vi "XLP80_Action_InitWriteB.vi"(8 "err in":errorcluster) -> (0 "err out":errorcluster)   [LabVIEW 2021]
uses:
  XLP80_State_V001.llb/XLP80_State_TDefEnumGlobalState.ctl
  XLP80_Globals/Globals_Settings_XLP80.vi
  XLP80_Globals/XLP80_Globals_Referenzen.vi
  XLP80_Globals/XLP80_CAN_Globals.vi
panel:
  out "Index HV&Software":i32[](array[numeric])
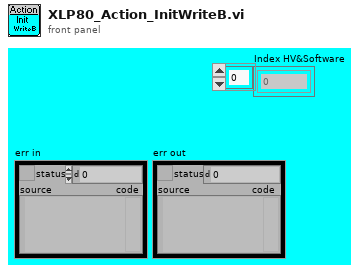
[diagram p1: front panel]
types:
  T1 = typedef "XLP80_State_TDefEnumGlobalState.ctl" = enum16{"HV & Software", "Basis Funktion", "Power Management", "Operational Mode", "Shutdown", "Alarm"}
  T2 = cluster{"Signal Name":string[], "Description":string[], "Unit":string[], "Default":dbl[], "Min":dbl[], "Max":dbl[], "Preconditions":bool[], "HV & Software":bool[], "Basis Funktion":bool[], "Power Management":bool[], "OperationMode":bool[], "Shutdown":bool[], "Alarm":bool[], "LogEnable":bool[]}
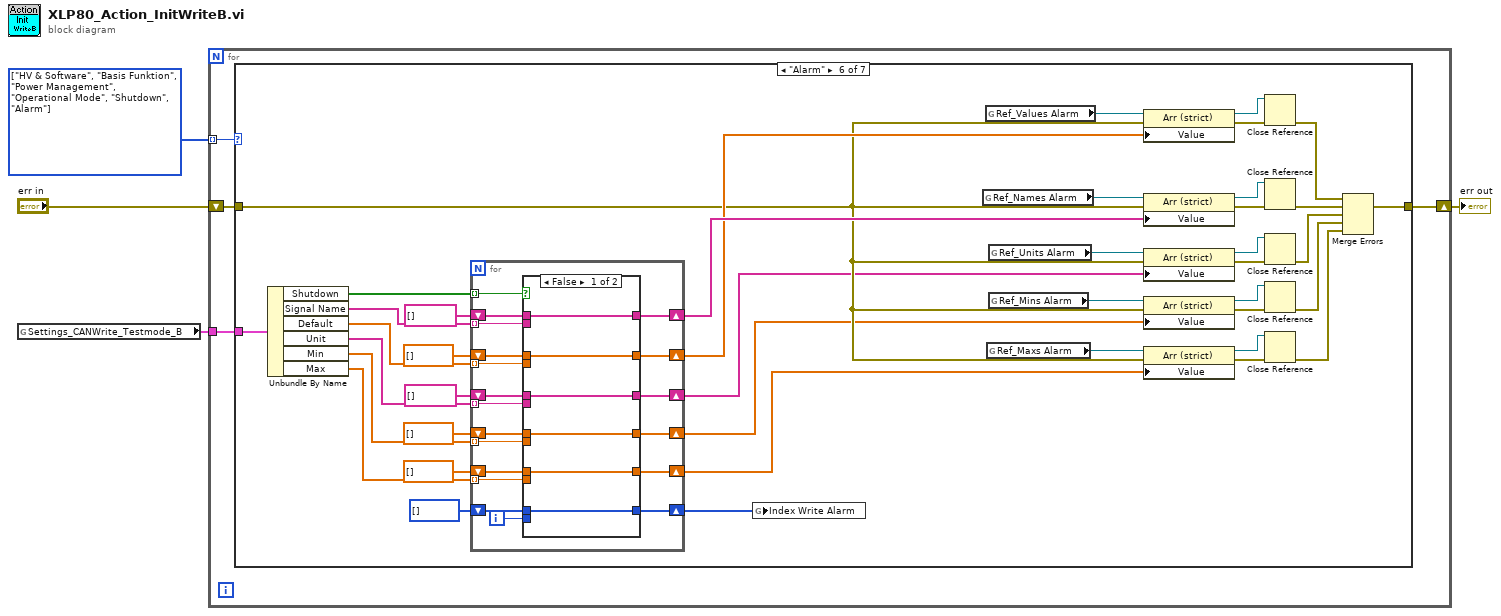
[diagram p0: block diagram]
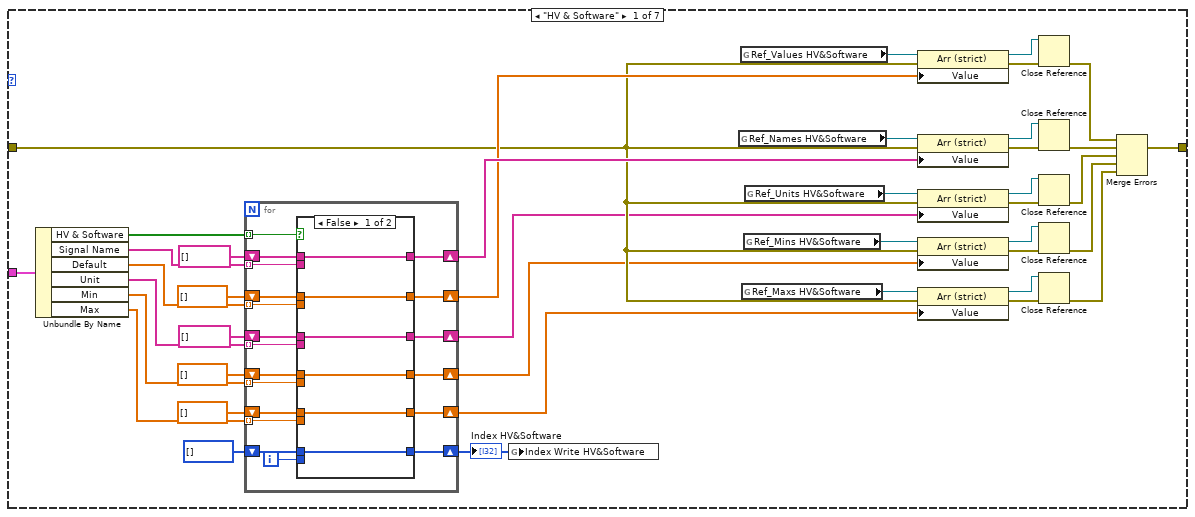
[diagram p2: hidden frame]
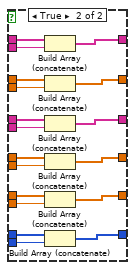
[diagram p3: hidden frame]
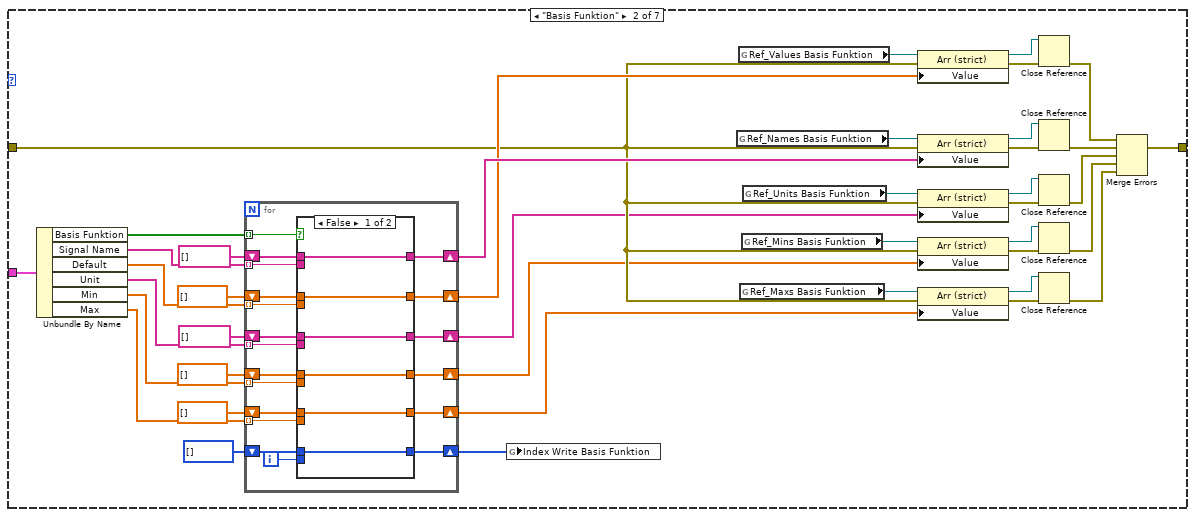
[diagram p4: hidden frame]
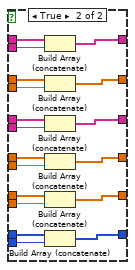
[diagram p5: hidden frame]
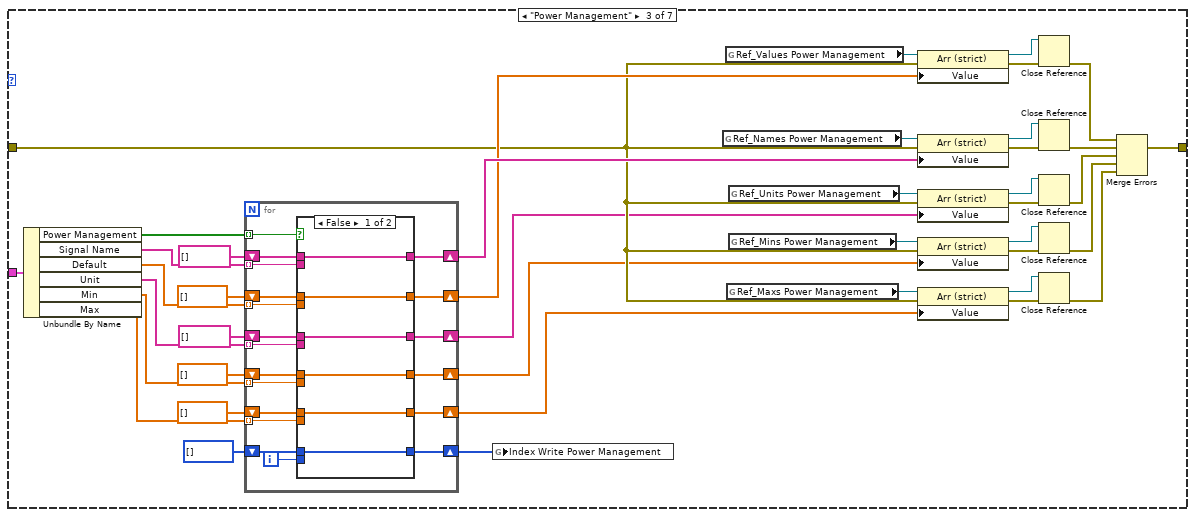
[diagram p6: hidden frame]
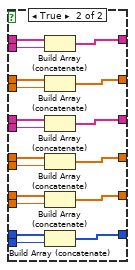
[diagram p7: hidden frame]
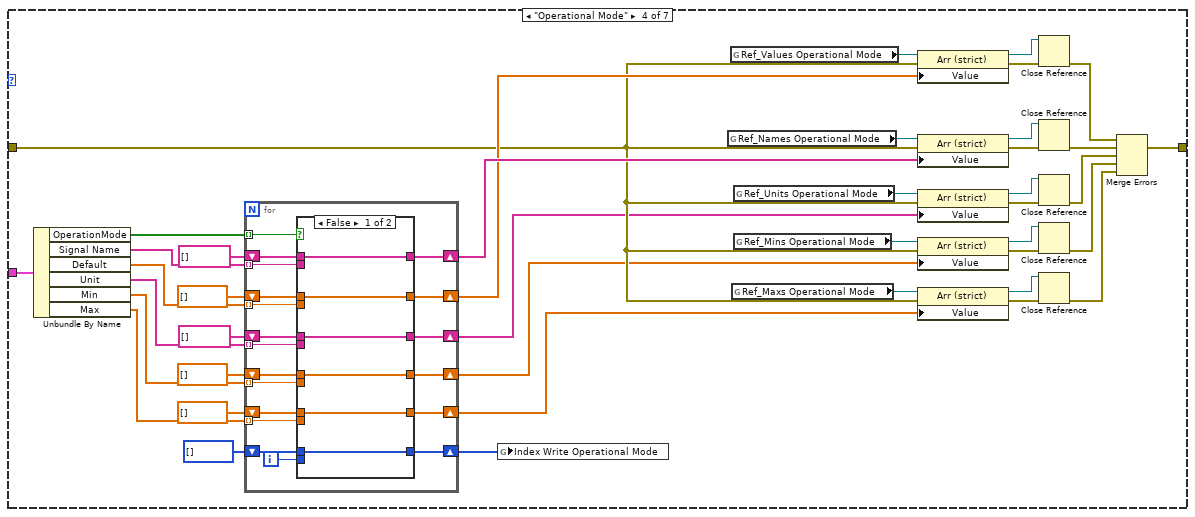
[diagram p8: hidden frame]
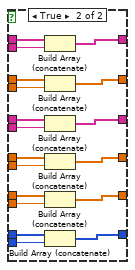
[diagram p9: hidden frame]
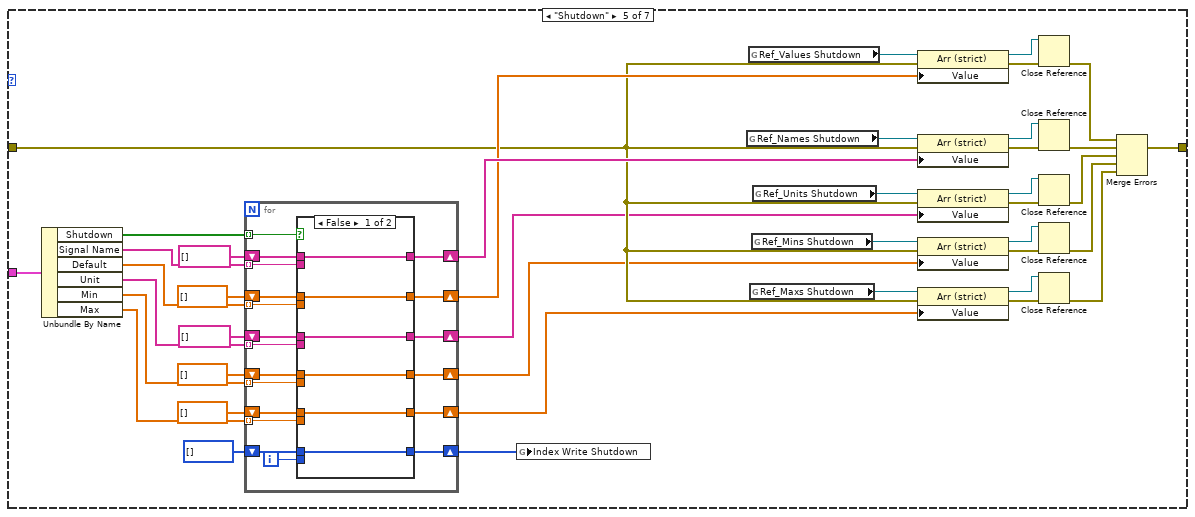
[diagram p10: hidden frame]
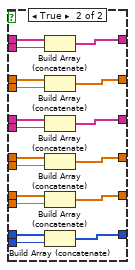
[diagram p11: hidden frame]
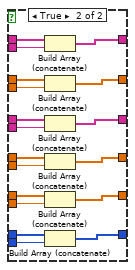
[diagram p12: hidden frame]
diagram:
  w1 = T1[] [enum."HV & Software", enum."Basis Funktion", enum."Power Management", enum."Operational Mode", enum."Shutdown", enum."Alarm"] items=["HV & Software", "Basis Funktion", "Power Management", "Operational Mode", "Shutdown", "Alarm"]
  n1 = global read "Globals_Settings_XLP80.vi" "Settings_CANWrite_Testmode_B"() -> (w4:T2)
  n2 = for {
    tunnel: w4 -> [w8]
    shift-right: [w6] -> w2
    shift-left: "err in" -> [w7]
    tunnel: w1 -> [w5] mode=indexing
    n3 = case shown="\"Alarm\"" w5 {
      tunnel: w8 -> [w49 w133 w217 w301 w385 w469 _]
      tunnel: w7 -> [w15 w99 w183 w267 w351 w435 w513]
      tunnel: [w35 w119 w203 w287 w371 w455 w513] -> w6
      frame "HV & Software" {
        n4 = Unbundle By Name(w49) -> ("HV & Software"=w40:bool[], "Signal Name"=w43:string[], "Default"=w32:dbl[], "Unit"=w27:string[], "Min"=w26:dbl[], "Max"=w25:dbl[])
        n5 = for {
          tunnel: w40 -> [w68] mode=indexing
          shift-right: [w65] -> w39
          shift-left: string[] [] ("Signal Name") -> [w67]
          shift-right: [w62] -> w41
          shift-left: i32[] [] -> [w64]
          tunnel: w43 -> [w66] mode=indexing
          shift-right: [w59] -> w31
          shift-left: dbl[] [] ("Default") -> [w61]
          tunnel: w32 -> [w60] mode=indexing
          shift-right: [w58] -> w10
          shift-left: dbl[] [] ("Default") -> [w56]
          tunnel: w26 -> [w57] mode=indexing
          shift-right: [w53] -> w9
          shift-left: dbl[] [] ("Default") -> [w55]
          tunnel: w25 -> [w54] mode=indexing
          shift-right: [w52] -> w11
          shift-left: string[] [] ("Signal Name") -> [w50]
          tunnel: w27 -> [w51] mode=indexing
          i -> [w63]
          n6 = case shown="False" w68 {
            tunnel: w67 -> [w74 w92]
            tunnel: w66 -> [_ w91]
            tunnel: [w74 w90] -> w65
            tunnel: w64 -> [w73 w89]
            tunnel: w63 -> [_ w88]
            tunnel: [w73 w87] -> w62
            tunnel: w61 -> [w72 w86]
            tunnel: w60 -> [_ w85]
            tunnel: [w72 w84] -> w59
            tunnel: w56 -> [w70 w81]
            tunnel: w57 -> [_ w82]
            tunnel: [w70 w83] -> w58
            tunnel: w55 -> [w69 w80]
            tunnel: w54 -> [_ w79]
            tunnel: [w69 w78] -> w53
            tunnel: w50 -> [w71 w75]
            tunnel: w51 -> [_ w76]
            tunnel: [w71 w77] -> w52
            frame False {
            }
            frame True {
              n7 = Build Array (concatenate)(w92, w91) -> (w90:string[])
              n8 = Build Array (concatenate)(w86, w85) -> (w84:dbl[])
              n9 = Build Array (concatenate)(w75, w76) -> (w77:string[])
              n10 = Build Array (concatenate)(w81, w82) -> (w83:dbl[])
              n11 = Build Array (concatenate)(w80, w79) -> (w78:dbl[])
              n12 = Build Array (concatenate)(w89, w88) -> (w87:i32[])
            }
          }
        }
        "Index HV&Software" <- w41
        n13 = global write "XLP80_CAN_Globals.vi" "Index Write HV&Software"(w41) -> ()
        n14 = global read "XLP80_Globals_Referenzen.vi" "Ref_Names HV&Software"() -> (w46:refnum<vi>)
        n15 = global read "XLP80_Globals_Referenzen.vi" "Ref_Values HV&Software"() -> (w36:refnum<vi>)
        n16 = global read "XLP80_Globals_Referenzen.vi" "Ref_Maxs HV&Software"() -> (w16:refnum<vi>)
        n17 = global read "XLP80_Globals_Referenzen.vi" "Ref_Mins HV&Software"() -> (w21:refnum<vi>)
        n18 = global read "XLP80_Globals_Referenzen.vi" "Ref_Units HV&Software"() -> (w24:refnum<vi>)
        n19 = property class="Arr (strict)"(reference=w36, error in=w15, "Value"=w31) -> (reference out=w38:refnum<vi>, error out=w37:errorcluster)
        n20 = property class="Arr (strict)"(reference=w46, error in=w15, "Value"=w39) -> (reference out=w47:refnum<vi>, error out=w48:errorcluster)
        n21 = property class="Arr (strict)"(reference=w24, error in=w15, "Value"=w11) -> (reference out=w22:refnum<vi>, error out=w23:errorcluster)
        n22 = property class="Arr (strict)"(reference=w21, error in=w15, "Value"=w10) -> (reference out=w20:refnum<vi>, error out=w19:errorcluster)
        n23 = property class="Arr (strict)"(reference=w16, error in=w15, "Value"=w9) -> (reference out=w17:refnum<vi>, error out=w18:errorcluster)
        n24 = Close Reference(reference=w38, error in (no error)=w37) -> (error out=w34:errorcluster)
        n25 = Close Reference(reference=w47, error in (no error)=w48) -> (error out=w45:errorcluster)
        n26 = Close Reference(reference=w22, error in (no error)=w23) -> (error out=w14:errorcluster)
        n27 = Close Reference(reference=w20, error in (no error)=w19) -> (error out=w13:errorcluster)
        n28 = Close Reference(reference=w17, error in (no error)=w18) -> (error out=w12:errorcluster)
        n29 = Merge Errors(w34, w45, w14, w13, w12) -> (w35:errorcluster)
      }
      frame "Basis Funktion" {
        n30 = Unbundle By Name(w133) -> ("Basis Funktion"=w124:bool[], "Signal Name"=w127:string[], "Default"=w116:dbl[], "Unit"=w111:string[], "Min"=w110:dbl[], "Max"=w109:dbl[])
        n31 = for {
          tunnel: w124 -> [w152] mode=indexing
          shift-right: [w149] -> w123
          shift-left: string[] [] ("Signal Name") -> [w151]
          shift-right: [w146] -> w125
          shift-left: i32[] [] -> [w148]
          tunnel: w127 -> [w150] mode=indexing
          shift-right: [w143] -> w115
          shift-left: dbl[] [] ("Default") -> [w145]
          tunnel: w116 -> [w144] mode=indexing
          shift-right: [w142] -> w94
          shift-left: dbl[] [] ("Default") -> [w140]
          tunnel: w110 -> [w141] mode=indexing
          shift-right: [w137] -> w93
          shift-left: dbl[] [] ("Default") -> [w139]
          tunnel: w109 -> [w138] mode=indexing
          shift-right: [w136] -> w95
          shift-left: string[] [] ("Signal Name") -> [w134]
          tunnel: w111 -> [w135] mode=indexing
          i -> [w147]
          n32 = case shown="False" w152 {
            tunnel: w151 -> [w158 w176]
            tunnel: w150 -> [_ w175]
            tunnel: [w158 w174] -> w149
            tunnel: w148 -> [w157 w173]
            tunnel: w147 -> [_ w172]
            tunnel: [w157 w171] -> w146
            tunnel: w145 -> [w156 w170]
            tunnel: w144 -> [_ w169]
            tunnel: [w156 w168] -> w143
            tunnel: w140 -> [w154 w165]
            tunnel: w141 -> [_ w166]
            tunnel: [w154 w167] -> w142
            tunnel: w139 -> [w153 w164]
            tunnel: w138 -> [_ w163]
            tunnel: [w153 w162] -> w137
            tunnel: w134 -> [w155 w159]
            tunnel: w135 -> [_ w160]
            tunnel: [w155 w161] -> w136
            frame False {
            }
            frame True {
              n33 = Build Array (concatenate)(w176, w175) -> (w174:string[])
              n34 = Build Array (concatenate)(w170, w169) -> (w168:dbl[])
              n35 = Build Array (concatenate)(w159, w160) -> (w161:string[])
              n36 = Build Array (concatenate)(w165, w166) -> (w167:dbl[])
              n37 = Build Array (concatenate)(w164, w163) -> (w162:dbl[])
              n38 = Build Array (concatenate)(w173, w172) -> (w171:i32[])
            }
          }
        }
        n39 = global write "XLP80_CAN_Globals.vi" "Index Write Basis Funktion"(w125) -> ()
        n40 = global read "XLP80_Globals_Referenzen.vi" "Ref_Names Basis Funktion"() -> (w130:refnum<vi>)
        n41 = global read "XLP80_Globals_Referenzen.vi" "Ref_Values Basis Funktion"() -> (w120:refnum<vi>)
        n42 = global read "XLP80_Globals_Referenzen.vi" "Ref_Maxs Basis Funktion"() -> (w100:refnum<vi>)
        n43 = global read "XLP80_Globals_Referenzen.vi" "Ref_Mins Basis Funktion"() -> (w105:refnum<vi>)
        n44 = global read "XLP80_Globals_Referenzen.vi" "Ref_Units Basis Funktion"() -> (w108:refnum<vi>)
        n45 = property class="Arr (strict)"(reference=w120, error in=w99, "Value"=w115) -> (reference out=w122:refnum<vi>, error out=w121:errorcluster)
        n46 = property class="Arr (strict)"(reference=w130, error in=w99, "Value"=w123) -> (reference out=w131:refnum<vi>, error out=w132:errorcluster)
        n47 = property class="Arr (strict)"(reference=w108, error in=w99, "Value"=w95) -> (reference out=w106:refnum<vi>, error out=w107:errorcluster)
        n48 = property class="Arr (strict)"(reference=w105, error in=w99, "Value"=w94) -> (reference out=w104:refnum<vi>, error out=w103:errorcluster)
        n49 = property class="Arr (strict)"(reference=w100, error in=w99, "Value"=w93) -> (reference out=w101:refnum<vi>, error out=w102:errorcluster)
        n50 = Close Reference(reference=w122, error in (no error)=w121) -> (error out=w118:errorcluster)
        n51 = Close Reference(reference=w131, error in (no error)=w132) -> (error out=w129:errorcluster)
        n52 = Close Reference(reference=w106, error in (no error)=w107) -> (error out=w98:errorcluster)
        n53 = Close Reference(reference=w104, error in (no error)=w103) -> (error out=w97:errorcluster)
        n54 = Close Reference(reference=w101, error in (no error)=w102) -> (error out=w96:errorcluster)
        n55 = Merge Errors(w118, w129, w98, w97, w96) -> (w119:errorcluster)
      }
      frame "Power Management" {
        n56 = Unbundle By Name(w217) -> ("Power Management"=w208:bool[], "Signal Name"=w211:string[], "Default"=w200:dbl[], "Unit"=w195:string[], "Min"=w194:dbl[], "Max"=w193:dbl[])
        n57 = for {
          tunnel: w208 -> [w236] mode=indexing
          shift-right: [w233] -> w207
          shift-left: string[] [] ("Signal Name") -> [w235]
          shift-right: [w230] -> w209
          shift-left: i32[] [] -> [w232]
          tunnel: w211 -> [w234] mode=indexing
          shift-right: [w227] -> w199
          shift-left: dbl[] [] ("Default") -> [w229]
          tunnel: w200 -> [w228] mode=indexing
          shift-right: [w226] -> w178
          shift-left: dbl[] [] ("Default") -> [w224]
          tunnel: w194 -> [w225] mode=indexing
          shift-right: [w221] -> w177
          shift-left: dbl[] [] ("Default") -> [w223]
          tunnel: w193 -> [w222] mode=indexing
          shift-right: [w220] -> w179
          shift-left: string[] [] ("Signal Name") -> [w218]
          tunnel: w195 -> [w219] mode=indexing
          i -> [w231]
          n58 = case shown="False" w236 {
            tunnel: w235 -> [w242 w260]
            tunnel: w234 -> [_ w259]
            tunnel: [w242 w258] -> w233
            tunnel: w232 -> [w241 w257]
            tunnel: w231 -> [_ w256]
            tunnel: [w241 w255] -> w230
            tunnel: w229 -> [w240 w254]
            tunnel: w228 -> [_ w253]
            tunnel: [w240 w252] -> w227
            tunnel: w224 -> [w238 w249]
            tunnel: w225 -> [_ w250]
            tunnel: [w238 w251] -> w226
            tunnel: w223 -> [w237 w248]
            tunnel: w222 -> [_ w247]
            tunnel: [w237 w246] -> w221
            tunnel: w218 -> [w239 w243]
            tunnel: w219 -> [_ w244]
            tunnel: [w239 w245] -> w220
            frame False {
            }
            frame True {
              n59 = Build Array (concatenate)(w260, w259) -> (w258:string[])
              n60 = Build Array (concatenate)(w254, w253) -> (w252:dbl[])
              n61 = Build Array (concatenate)(w243, w244) -> (w245:string[])
              n62 = Build Array (concatenate)(w249, w250) -> (w251:dbl[])
              n63 = Build Array (concatenate)(w248, w247) -> (w246:dbl[])
              n64 = Build Array (concatenate)(w257, w256) -> (w255:i32[])
            }
          }
        }
        n65 = global write "XLP80_CAN_Globals.vi" "Index Write Power Management"(w209) -> ()
        n66 = global read "XLP80_Globals_Referenzen.vi" "Ref_Names Power Management"() -> (w214:refnum<vi>)
        n67 = global read "XLP80_Globals_Referenzen.vi" "Ref_Values Power Management"() -> (w204:refnum<vi>)
        n68 = global read "XLP80_Globals_Referenzen.vi" "Ref_Maxs Power Management"() -> (w184:refnum<vi>)
        n69 = global read "XLP80_Globals_Referenzen.vi" "Ref_Units Power Management"() -> (w192:refnum<vi>)
        n70 = global read "XLP80_Globals_Referenzen.vi" "Ref_Mins Power Management"() -> (w189:refnum<vi>)
        n71 = property class="Arr (strict)"(reference=w204, error in=w183, "Value"=w199) -> (reference out=w206:refnum<vi>, error out=w205:errorcluster)
        n72 = property class="Arr (strict)"(reference=w214, error in=w183, "Value"=w207) -> (reference out=w215:refnum<vi>, error out=w216:errorcluster)
        n73 = property class="Arr (strict)"(reference=w192, error in=w183, "Value"=w179) -> (reference out=w190:refnum<vi>, error out=w191:errorcluster)
        n74 = property class="Arr (strict)"(reference=w189, error in=w183, "Value"=w178) -> (reference out=w188:refnum<vi>, error out=w187:errorcluster)
        n75 = property class="Arr (strict)"(reference=w184, error in=w183, "Value"=w177) -> (reference out=w185:refnum<vi>, error out=w186:errorcluster)
        n76 = Close Reference(reference=w206, error in (no error)=w205) -> (error out=w202:errorcluster)
        n77 = Close Reference(reference=w215, error in (no error)=w216) -> (error out=w213:errorcluster)
        n78 = Close Reference(reference=w190, error in (no error)=w191) -> (error out=w182:errorcluster)
        n79 = Close Reference(reference=w188, error in (no error)=w187) -> (error out=w181:errorcluster)
        n80 = Close Reference(reference=w185, error in (no error)=w186) -> (error out=w180:errorcluster)
        n81 = Merge Errors(w202, w213, w182, w181, w180) -> (w203:errorcluster)
      }
      frame "Operational Mode" {
        n82 = Unbundle By Name(w301) -> ("OperationMode"=w292:bool[], "Signal Name"=w295:string[], "Default"=w284:dbl[], "Unit"=w279:string[], "Min"=w278:dbl[], "Max"=w277:dbl[])
        n83 = for {
          tunnel: w292 -> [w320] mode=indexing
          shift-right: [w317] -> w291
          shift-left: string[] [] ("Signal Name") -> [w319]
          shift-right: [w314] -> w293
          shift-left: i32[] [] -> [w316]
          tunnel: w295 -> [w318] mode=indexing
          shift-right: [w311] -> w283
          shift-left: dbl[] [] ("Default") -> [w313]
          tunnel: w284 -> [w312] mode=indexing
          shift-right: [w310] -> w262
          shift-left: dbl[] [] ("Default") -> [w308]
          tunnel: w278 -> [w309] mode=indexing
          shift-right: [w305] -> w261
          shift-left: dbl[] [] ("Default") -> [w307]
          tunnel: w277 -> [w306] mode=indexing
          shift-right: [w304] -> w263
          shift-left: string[] [] ("Signal Name") -> [w302]
          tunnel: w279 -> [w303] mode=indexing
          i -> [w315]
          n84 = case shown="False" w320 {
            tunnel: w319 -> [w326 w344]
            tunnel: w318 -> [_ w343]
            tunnel: [w326 w342] -> w317
            tunnel: w316 -> [w325 w341]
            tunnel: w315 -> [_ w340]
            tunnel: [w325 w339] -> w314
            tunnel: w313 -> [w324 w338]
            tunnel: w312 -> [_ w337]
            tunnel: [w324 w336] -> w311
            tunnel: w308 -> [w322 w333]
            tunnel: w309 -> [_ w334]
            tunnel: [w322 w335] -> w310
            tunnel: w307 -> [w321 w332]
            tunnel: w306 -> [_ w331]
            tunnel: [w321 w330] -> w305
            tunnel: w302 -> [w323 w327]
            tunnel: w303 -> [_ w328]
            tunnel: [w323 w329] -> w304
            frame False {
            }
            frame True {
              n85 = Build Array (concatenate)(w344, w343) -> (w342:string[])
              n86 = Build Array (concatenate)(w338, w337) -> (w336:dbl[])
              n87 = Build Array (concatenate)(w327, w328) -> (w329:string[])
              n88 = Build Array (concatenate)(w333, w334) -> (w335:dbl[])
              n89 = Build Array (concatenate)(w332, w331) -> (w330:dbl[])
              n90 = Build Array (concatenate)(w341, w340) -> (w339:i32[])
            }
          }
        }
        n91 = global write "XLP80_CAN_Globals.vi" "Index Write Operational Mode"(w293) -> ()
        n92 = global read "XLP80_Globals_Referenzen.vi" "Ref_Names Operational Mode"() -> (w298:refnum<vi>)
        n93 = global read "XLP80_Globals_Referenzen.vi" "Ref_Values Operational Mode"() -> (w288:refnum<vi>)
        n94 = global read "XLP80_Globals_Referenzen.vi" "Ref_Maxs Operational Mode"() -> (w268:refnum<vi>)
        n95 = global read "XLP80_Globals_Referenzen.vi" "Ref_Units Operational Mode"() -> (w276:refnum<vi>)
        n96 = global read "XLP80_Globals_Referenzen.vi" "Ref_Mins Operational Mode"() -> (w273:refnum<vi>)
        n97 = property class="Arr (strict)"(reference=w288, error in=w267, "Value"=w283) -> (reference out=w290:refnum<vi>, error out=w289:errorcluster)
        n98 = property class="Arr (strict)"(reference=w298, error in=w267, "Value"=w291) -> (reference out=w299:refnum<vi>, error out=w300:errorcluster)
        n99 = property class="Arr (strict)"(reference=w276, error in=w267, "Value"=w263) -> (reference out=w274:refnum<vi>, error out=w275:errorcluster)
        n100 = property class="Arr (strict)"(reference=w273, error in=w267, "Value"=w262) -> (reference out=w272:refnum<vi>, error out=w271:errorcluster)
        n101 = property class="Arr (strict)"(reference=w268, error in=w267, "Value"=w261) -> (reference out=w269:refnum<vi>, error out=w270:errorcluster)
        n102 = Close Reference(reference=w290, error in (no error)=w289) -> (error out=w286:errorcluster)
        n103 = Close Reference(reference=w299, error in (no error)=w300) -> (error out=w297:errorcluster)
        n104 = Close Reference(reference=w274, error in (no error)=w275) -> (error out=w266:errorcluster)
        n105 = Close Reference(reference=w272, error in (no error)=w271) -> (error out=w265:errorcluster)
        n106 = Close Reference(reference=w269, error in (no error)=w270) -> (error out=w264:errorcluster)
        n107 = Merge Errors(w286, w297, w266, w265, w264) -> (w287:errorcluster)
      }
      frame "Shutdown" {
        n108 = Unbundle By Name(w385) -> ("Shutdown"=w376:bool[], "Signal Name"=w379:string[], "Default"=w368:dbl[], "Unit"=w363:string[], "Min"=w362:dbl[], "Max"=w361:dbl[])
        n109 = for {
          tunnel: w376 -> [w404] mode=indexing
          shift-right: [w401] -> w375
          shift-left: string[] [] ("Signal Name") -> [w403]
          shift-right: [w398] -> w377
          shift-left: i32[] [] -> [w400]
          tunnel: w379 -> [w402] mode=indexing
          shift-right: [w395] -> w367
          shift-left: dbl[] [] ("Default") -> [w397]
          tunnel: w368 -> [w396] mode=indexing
          shift-right: [w394] -> w346
          shift-left: dbl[] [] ("Default") -> [w392]
          tunnel: w362 -> [w393] mode=indexing
          shift-right: [w389] -> w345
          shift-left: dbl[] [] ("Default") -> [w391]
          tunnel: w361 -> [w390] mode=indexing
          shift-right: [w388] -> w347
          shift-left: string[] [] ("Signal Name") -> [w386]
          tunnel: w363 -> [w387] mode=indexing
          i -> [w399]
          n110 = case shown="False" w404 {
            tunnel: w403 -> [w410 w428]
            tunnel: w402 -> [_ w427]
            tunnel: [w410 w426] -> w401
            tunnel: w400 -> [w409 w425]
            tunnel: w399 -> [_ w424]
            tunnel: [w409 w423] -> w398
            tunnel: w397 -> [w408 w422]
            tunnel: w396 -> [_ w421]
            tunnel: [w408 w420] -> w395
            tunnel: w392 -> [w406 w417]
            tunnel: w393 -> [_ w418]
            tunnel: [w406 w419] -> w394
            tunnel: w391 -> [w405 w416]
            tunnel: w390 -> [_ w415]
            tunnel: [w405 w414] -> w389
            tunnel: w386 -> [w407 w411]
            tunnel: w387 -> [_ w412]
            tunnel: [w407 w413] -> w388
            frame False {
            }
            frame True {
              n111 = Build Array (concatenate)(w428, w427) -> (w426:string[])
              n112 = Build Array (concatenate)(w422, w421) -> (w420:dbl[])
              n113 = Build Array (concatenate)(w411, w412) -> (w413:string[])
              n114 = Build Array (concatenate)(w417, w418) -> (w419:dbl[])
              n115 = Build Array (concatenate)(w416, w415) -> (w414:dbl[])
              n116 = Build Array (concatenate)(w425, w424) -> (w423:i32[])
            }
          }
        }
        n117 = global write "XLP80_CAN_Globals.vi" "Index Write Shutdown"(w377) -> ()
        n118 = global read "XLP80_Globals_Referenzen.vi" "Ref_Names Shutdown"() -> (w382:refnum<vi>)
        n119 = global read "XLP80_Globals_Referenzen.vi" "Ref_Values Shutdown"() -> (w372:refnum<vi>)
        n120 = global read "XLP80_Globals_Referenzen.vi" "Ref_Maxs Shutdown"() -> (w352:refnum<vi>)
        n121 = global read "XLP80_Globals_Referenzen.vi" "Ref_Mins Shutdown"() -> (w357:refnum<vi>)
        n122 = global read "XLP80_Globals_Referenzen.vi" "Ref_Units Shutdown"() -> (w360:refnum<vi>)
        n123 = property class="Arr (strict)"(reference=w372, error in=w351, "Value"=w367) -> (reference out=w374:refnum<vi>, error out=w373:errorcluster)
        n124 = property class="Arr (strict)"(reference=w382, error in=w351, "Value"=w375) -> (reference out=w383:refnum<vi>, error out=w384:errorcluster)
        n125 = property class="Arr (strict)"(reference=w360, error in=w351, "Value"=w347) -> (reference out=w358:refnum<vi>, error out=w359:errorcluster)
        n126 = property class="Arr (strict)"(reference=w357, error in=w351, "Value"=w346) -> (reference out=w356:refnum<vi>, error out=w355:errorcluster)
        n127 = property class="Arr (strict)"(reference=w352, error in=w351, "Value"=w345) -> (reference out=w353:refnum<vi>, error out=w354:errorcluster)
        n128 = Close Reference(reference=w374, error in (no error)=w373) -> (error out=w370:errorcluster)
        n129 = Close Reference(reference=w383, error in (no error)=w384) -> (error out=w381:errorcluster)
        n130 = Close Reference(reference=w358, error in (no error)=w359) -> (error out=w350:errorcluster)
        n131 = Close Reference(reference=w356, error in (no error)=w355) -> (error out=w349:errorcluster)
        n132 = Close Reference(reference=w353, error in (no error)=w354) -> (error out=w348:errorcluster)
        n133 = Merge Errors(w370, w381, w350, w349, w348) -> (w371:errorcluster)
      }
      frame "Alarm" {
        n134 = Unbundle By Name(w469) -> ("Shutdown"=w460:bool[], "Signal Name"=w463:string[], "Default"=w452:dbl[], "Unit"=w447:string[], "Min"=w446:dbl[], "Max"=w445:dbl[])
        n135 = for {
          tunnel: w460 -> [w488] mode=indexing
          shift-right: [w485] -> w459
          shift-left: string[] [] ("Signal Name") -> [w487]
          shift-right: [w482] -> w461
          shift-left: i32[] [] -> [w484]
          tunnel: w463 -> [w486] mode=indexing
          shift-right: [w479] -> w451
          shift-left: dbl[] [] ("Default") -> [w481]
          tunnel: w452 -> [w480] mode=indexing
          shift-right: [w478] -> w430
          shift-left: dbl[] [] ("Default") -> [w476]
          tunnel: w446 -> [w477] mode=indexing
          shift-right: [w473] -> w429
          shift-left: dbl[] [] ("Default") -> [w475]
          tunnel: w445 -> [w474] mode=indexing
          shift-right: [w472] -> w431
          shift-left: string[] [] ("Signal Name") -> [w470]
          tunnel: w447 -> [w471] mode=indexing
          i -> [w483]
          n136 = case shown="False" w488 {
            tunnel: w487 -> [w494 w512]
            tunnel: w486 -> [_ w511]
            tunnel: [w494 w510] -> w485
            tunnel: w484 -> [w493 w509]
            tunnel: w483 -> [_ w508]
            tunnel: [w493 w507] -> w482
            tunnel: w481 -> [w492 w506]
            tunnel: w480 -> [_ w505]
            tunnel: [w492 w504] -> w479
            tunnel: w476 -> [w490 w501]
            tunnel: w477 -> [_ w502]
            tunnel: [w490 w503] -> w478
            tunnel: w475 -> [w489 w500]
            tunnel: w474 -> [_ w499]
            tunnel: [w489 w498] -> w473
            tunnel: w470 -> [w491 w495]
            tunnel: w471 -> [_ w496]
            tunnel: [w491 w497] -> w472
            frame False {
            }
            frame True {
              n137 = Build Array (concatenate)(w512, w511) -> (w510:string[])
              n138 = Build Array (concatenate)(w506, w505) -> (w504:dbl[])
              n139 = Build Array (concatenate)(w495, w496) -> (w497:string[])
              n140 = Build Array (concatenate)(w501, w502) -> (w503:dbl[])
              n141 = Build Array (concatenate)(w500, w499) -> (w498:dbl[])
              n142 = Build Array (concatenate)(w509, w508) -> (w507:i32[])
            }
          }
        }
        n143 = global write "XLP80_CAN_Globals.vi" "Index Write Alarm"(w461) -> ()
        n144 = global read "XLP80_Globals_Referenzen.vi" "Ref_Names Alarm"() -> (w466:refnum<vi>)
        n145 = global read "XLP80_Globals_Referenzen.vi" "Ref_Values Alarm"() -> (w456:refnum<vi>)
        n146 = global read "XLP80_Globals_Referenzen.vi" "Ref_Maxs Alarm"() -> (w436:refnum<vi>)
        n147 = global read "XLP80_Globals_Referenzen.vi" "Ref_Units Alarm"() -> (w444:refnum<vi>)
        n148 = global read "XLP80_Globals_Referenzen.vi" "Ref_Mins Alarm"() -> (w441:refnum<vi>)
        n149 = property class="Arr (strict)"(reference=w456, error in=w435, "Value"=w451) -> (reference out=w458:refnum<vi>, error out=w457:errorcluster)
        n150 = property class="Arr (strict)"(reference=w466, error in=w435, "Value"=w459) -> (reference out=w467:refnum<vi>, error out=w468:errorcluster)
        n151 = property class="Arr (strict)"(reference=w444, error in=w435, "Value"=w431) -> (reference out=w442:refnum<vi>, error out=w443:errorcluster)
        n152 = property class="Arr (strict)"(reference=w441, error in=w435, "Value"=w430) -> (reference out=w440:refnum<vi>, error out=w439:errorcluster)
        n153 = property class="Arr (strict)"(reference=w436, error in=w435, "Value"=w429) -> (reference out=w437:refnum<vi>, error out=w438:errorcluster)
        n154 = Close Reference(reference=w458, error in (no error)=w457) -> (error out=w454:errorcluster)
        n155 = Close Reference(reference=w467, error in (no error)=w468) -> (error out=w465:errorcluster)
        n156 = Close Reference(reference=w442, error in (no error)=w443) -> (error out=w434:errorcluster)
        n157 = Close Reference(reference=w440, error in (no error)=w439) -> (error out=w433:errorcluster)
        n158 = Close Reference(reference=w437, error in (no error)=w438) -> (error out=w432:errorcluster)
        n159 = Merge Errors(w454, w465, w434, w433, w432) -> (w455:errorcluster)
      }
      frame Default {
      }
    }
  }
  "err out" <- w2
